vi "Cargo Intake TeleOp.vi"(11 "Controller Values":T1) -> ()   [LabVIEW 2018]
uses:
  Support Code/Controller Values.ctl
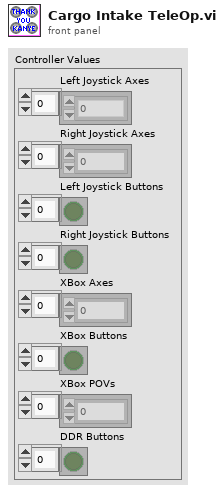
[diagram p1: front panel]
types:
  T1 = typedef "Controller Values.ctl" = cluster{"Left Joystick Axes ":dbl[], "Right Joystick Axes":dbl[], "Left Joystick Buttons":bool[], "Right Joystick Buttons":bool[], "XBox Axes":dbl[], "XBox Buttons":bool[], "XBox POVs":i16[], "DDR Buttons":bool[]}
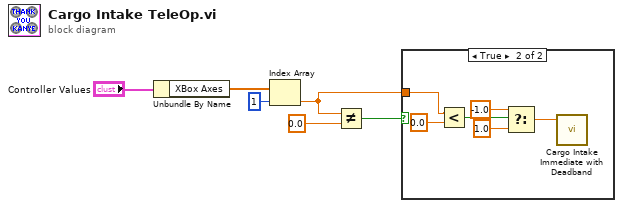
[diagram p0: block diagram]
diagram:
  n1 = Unbundle By Name("Controller Values") -> ("XBox Axes"=w1:dbl[])
  n2 = Index Array(array=w1, index=1) -> (element=w3:dbl)
  n3 = Not Equal?(x=w3, y=0.0) -> (x != y?=w4:bool)
  n4 = case shown="True" w4 {
    tunnel: w3 -> [_ w11]
    frame False {
    }
    frame True {
      n5 = Less?(x=w11, y=0.0) -> (x < y?=w12:bool)
      n6 = Select(t=-1.0, s=w12, f=1.0) -> (s? t:f=w7:dbl)
      n7 = call "Cargo Intake Immediate with Deadband.vi"("Setpoint"=w7) -> ()  [unwired: 10 in, 1 out]
    }
  }
